vi "D.vi"(2 "D":bool, 3 "R":bool, 4 "C":bool) -> (0 "~Q":bool, 1 "Q":bool)   [LabVIEW 2019, in "Triggers.lvlib"]
uses:
  Triggers.lvlib
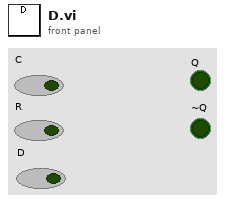
[diagram p1: front panel]
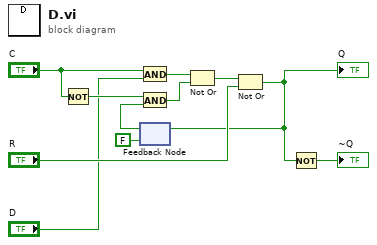
[diagram p0: block diagram]
diagram:
  n1 = Not(x="C") -> (.not. x?=w11:bool)
  n2 = And(x="C", y="D") -> (x .and. y?=w9:bool)
  n3 = feedback #1(FALSE) -> (w10:bool)
  n4 = And(x=w11, y=w10) -> (x .and. y?=w8:bool)
  n5 = Not Or(1:w8, 2:w9) -> (0:w7:bool)
  n6 = Not Or(1:"R", 2:w7) -> (0:w3:bool)
  "Q" <- w3
  n7 = feedback-in #1(w3) -> ()
  n8 = Not(x=w3) -> (.not. x?=→"~Q":bool)
